vi "Average.vi"(11 "Input":dbl) -> (3 "Average":dbl)   [LabVIEW 2011]
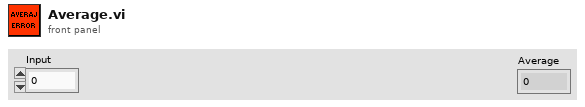
[diagram p1: front panel]
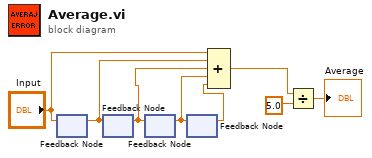
[diagram p0: block diagram]
diagram:
  n1 = feedback #1() -> (w5:dbl)  [unwired: 1 in]
  n2 = feedback-in #1("Input") -> ()
  n3 = feedback #2() -> (w4:dbl)  [unwired: 1 in]
  n4 = feedback-in #2(w5) -> ()
  n5 = feedback #3() -> (w3:dbl)  [unwired: 1 in]
  n6 = feedback-in #3(w4) -> ()
  n7 = feedback #4() -> (w2:dbl)  [unwired: 1 in]
  n8 = feedback-in #4(w3) -> ()
  n9 = Compound Arithmetic op=ADD("Input", w5, w4, w3, w2) -> (w1:dbl)
  n10 = Divide(x=w1, y=5.0) -> (x/y=→"Average":dbl)
